vi "6_AC_Akım_Harmonik.vi"(9 "Ölçüm Süresi [sn]":i32=60, 10 "Remote IP Address":string="10.1.21.100") -> (0 "error out":errorcluster, 1 "FD 2":dbl[][](array[numeric]) format="%_5f", 2 "FD 1":dbl[][](array[numeric]) format="%_5f")   [LabVIEW 2014]
panel:
  out "Akım Harmonik FD2 Ich":sgl[][](array[numeric]) format="%_5f"
  out "Akım Harmonik FD2 Ibh":sgl[][](array[numeric]) format="%_5f"
  out "Akım Harmonik FD2 Iah":sgl[][](array[numeric]) format="%_5f"
  in  "Akım Harmonik FD2 Ich Register":u16=1229
  in  "Akım Harmonik FD2 Ibh Register":u16=1129
  in  "Akım Harmonik FD2 Iah Register":u16=1029
  out "Akım Harmonik FD1 Ich":sgl[][](array[numeric]) format="%_5f"
  in  "Akım Harmonik FD1 Ich Register":u16=565
  out "Akım Harmonik FD1 Ibh":sgl[][](array[numeric]) format="%_5f"
  in  "Akım Harmonik FD1 Ibh Register":u16=465
  out "Akım Harmonik FD1 Iah":sgl[][](array[numeric]) format="%.4f"
  out "Numeric":i32
  in  "Akım Harmonik FD1 Iah Register":u16=365
  out "time stamp":timestamp=timestamp(1426515300 s since 1904-01-01) format="%<%H:%M:%S>T"
  in  "Remote Port":u16=1502
  in  "Stop":bool
  # "MB Ethernet Example Master.vi\n\nInstructions\n1. Run MB Ethernet Example Slave.vi\n2. Run this VI.\n3. Modify the discrete inputs or input registers on the slave -> they're updated on the master.\n4. Modify the coils and registers on the master -> they're updated on the slave."
  # "TCP Parameters"
  # "Slave Read-only Registers"
  # "1Har"
  # "1.Har"
  # "2.Har"
  # "3.Har"
  # "4.Har"
  # "5.Har"
  # "6.Har"
  # "7.Har"
  # "8.Har"
  # "9.Har"
  # "10.Har"
  # "2.Har"
  # "3.Har"
  # "4.Har"
  # "1Har"
  # "2.Har"
  # "3.Har"
  # "4.Har"
  # "1.Har"
  # "2.Har"
  # "3.Har"
  # "4.Har"
  # "5.Har"
  # "6.Har"
  # "7.Har"
  # "8.Har"
  # "9.Har"
  # "10.Har"
  # "1Har"
  # "2.Har"
  # "3.Har"
  # "4.Har"
  # "1Har"
  # "2.Har"
  # "3.Har"
  # "4.Har"
  # "1Har"
  # "2.Har"
  # "3.Har"
  # "4.Har"
  # "1Har"
  # "2.Har"
  # "3.Har"
  # "4.Har"
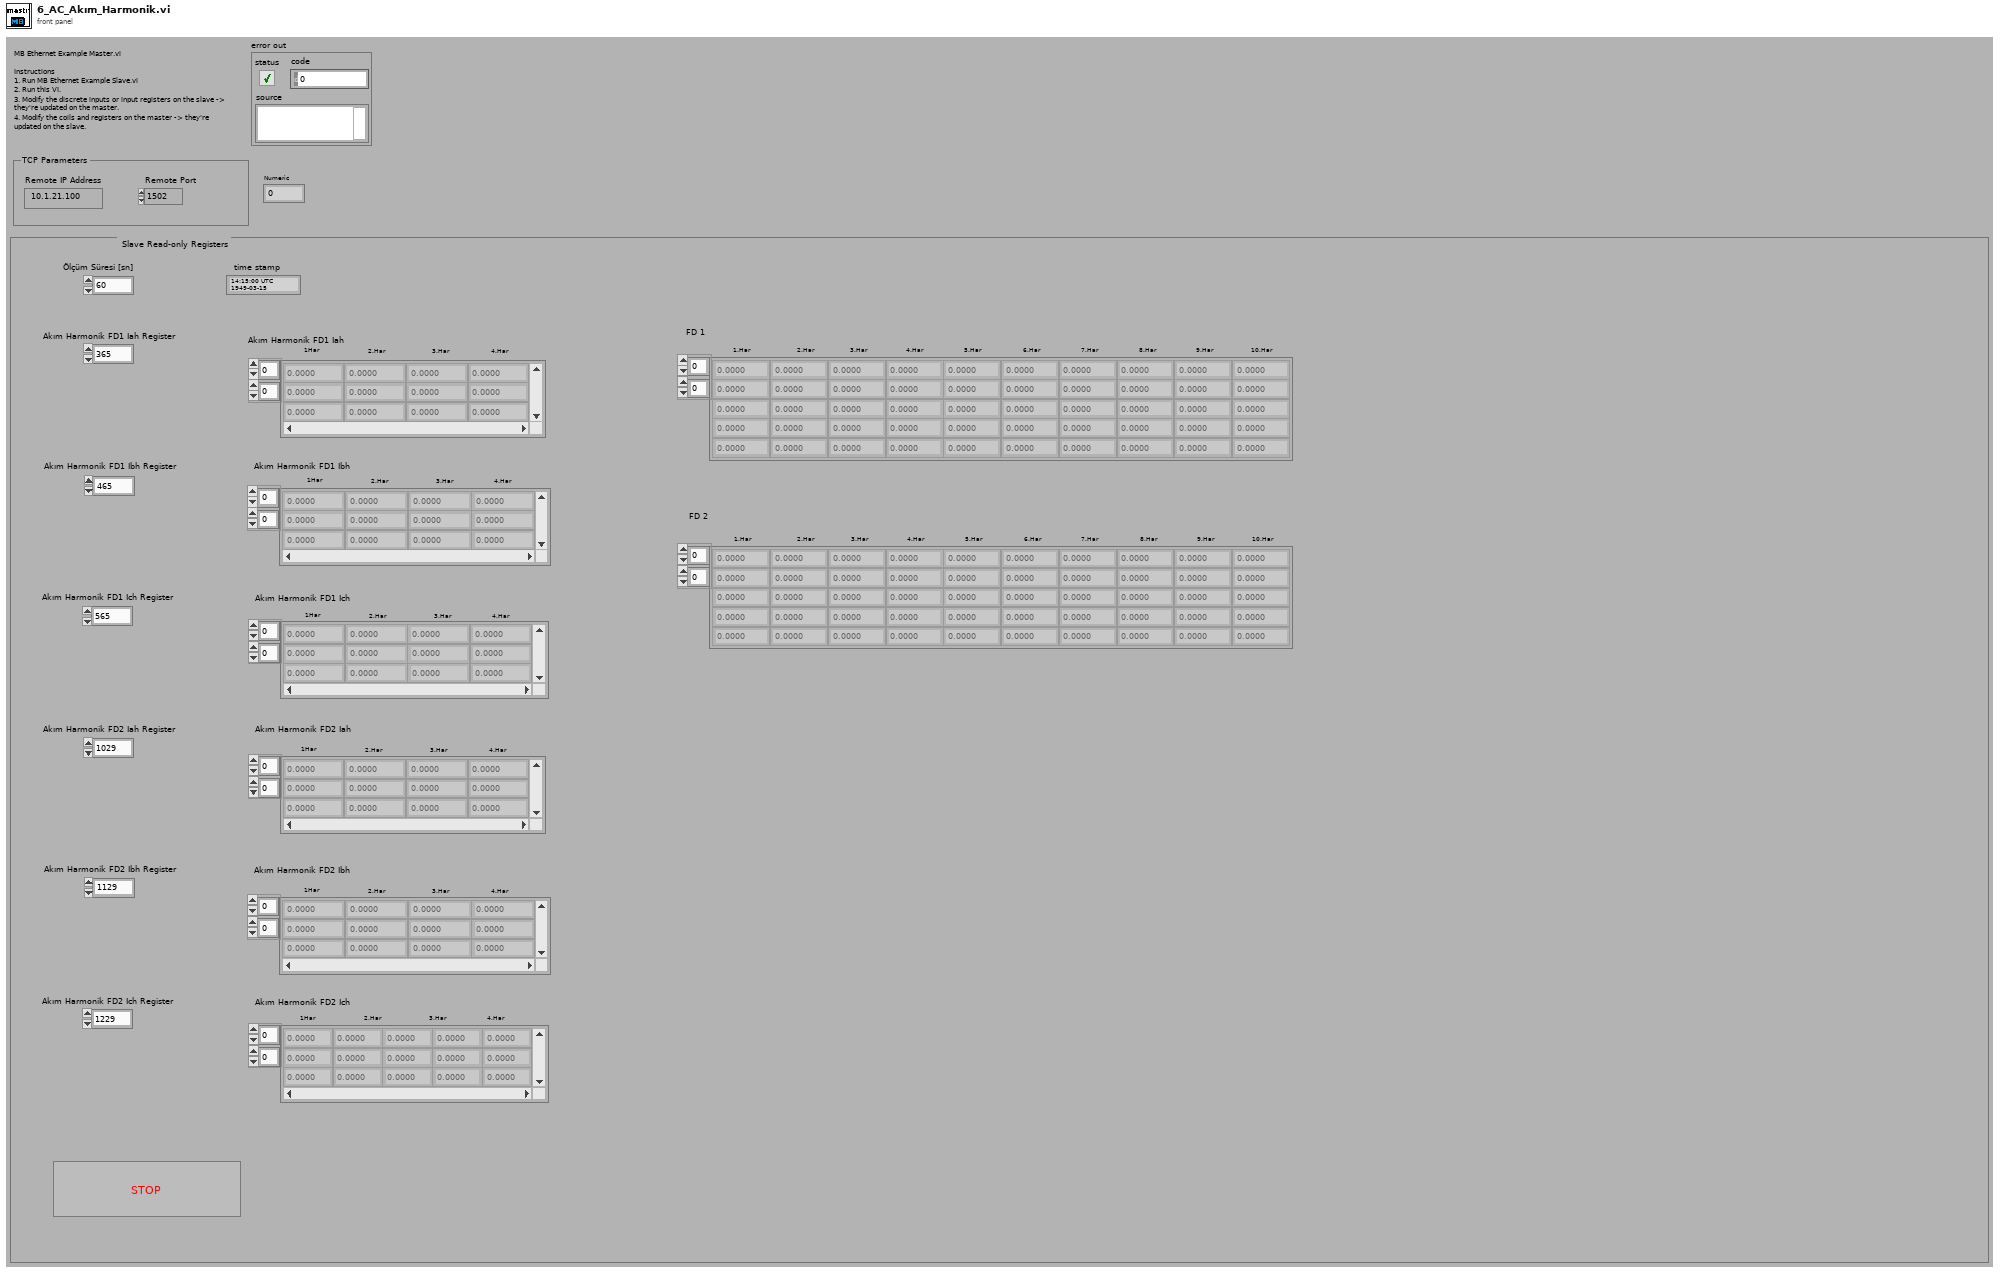
[diagram p1: front panel]
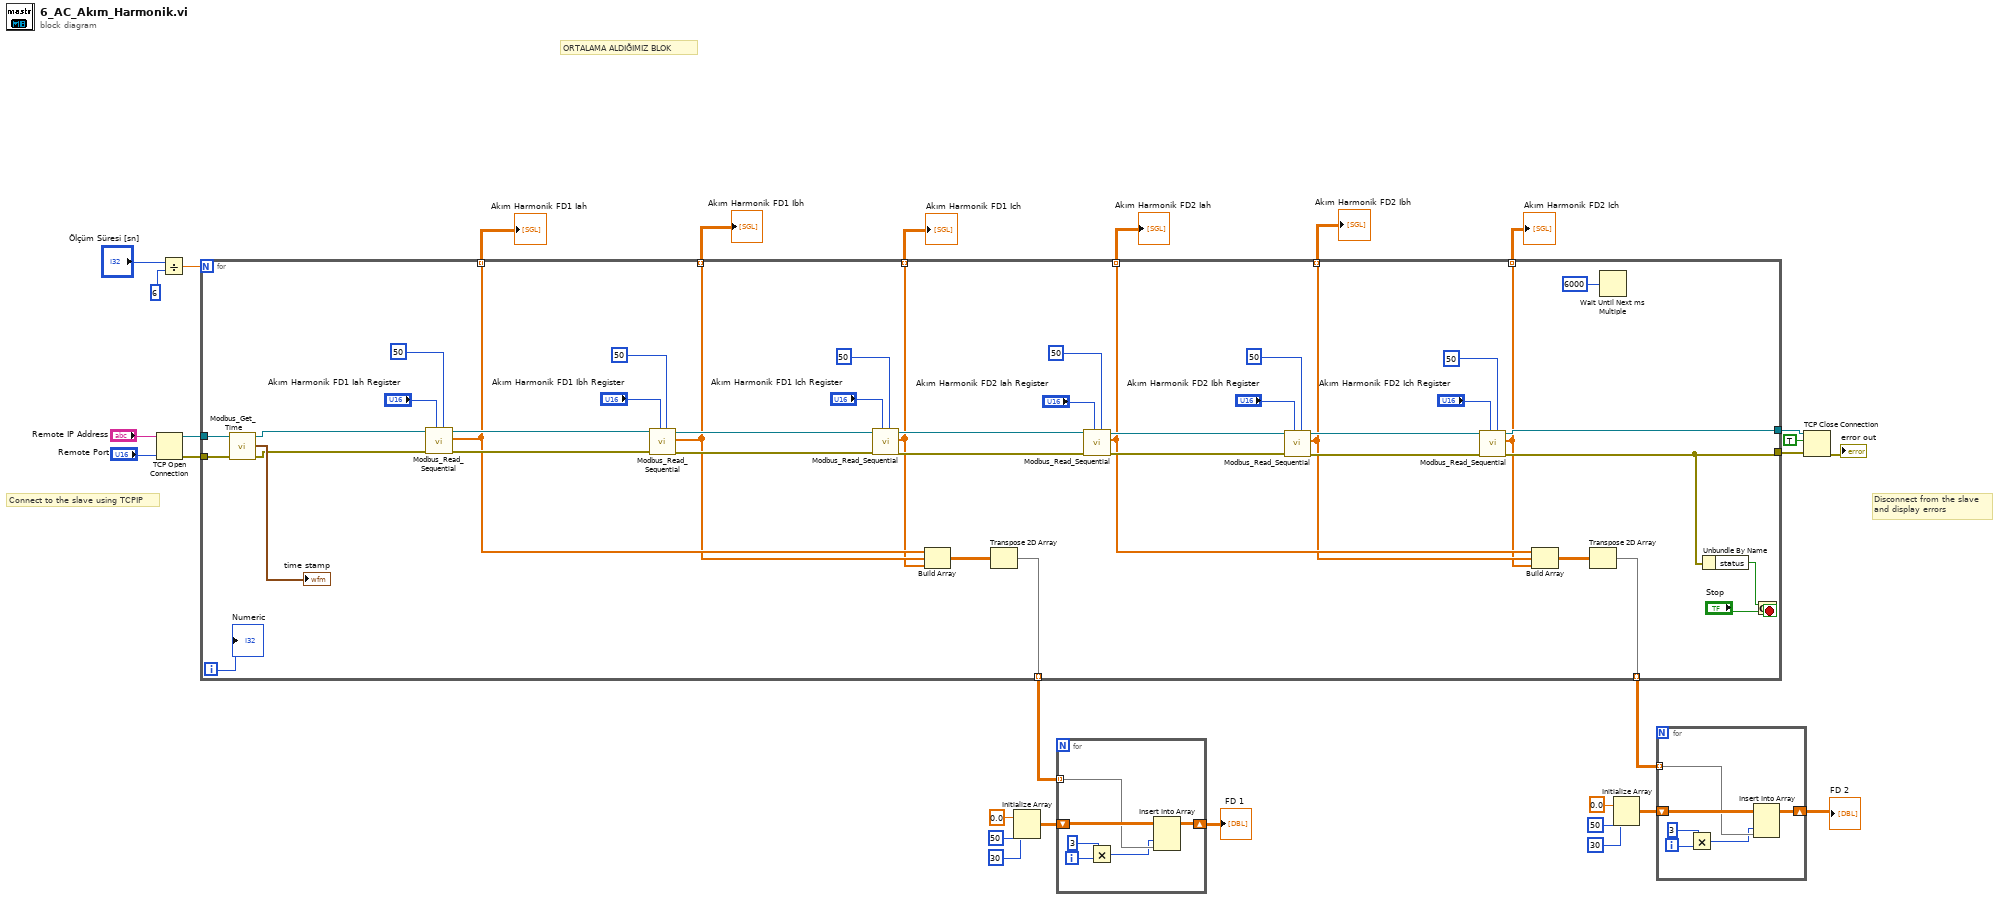
[diagram p0: block diagram]
diagram:
  # "ORTALAMA ALDIĞIMIZ BLOK"
  # "Disconnect from the slave\nand display errors"
  # "Connect to the slave using TCPIP"
  n1 = TCP Open Connection(address="Remote IP Address", remote port or service name="Remote Port") -> (connection ID=w27:refnum<k5>, error out=w26:errorcluster)  [unwired: 1 in, 2 out]
  n2 = Divide(x="Ölçüm Süresi [sn]", y=6) -> (x/y=w23:dbl)
  n3 = for {
    N: w23 -> [_]
    tunnel: w27 -> [w72]
    tunnel: w26 -> [w71]
    tunnel: [w39] -> w20 mode=indexing
    tunnel: [w38] -> w19 mode=indexing
    tunnel: [w37] -> w18 mode=indexing
    tunnel: [w36] -> w17 mode=indexing
    tunnel: [w35] -> w16 mode=indexing
    tunnel: [w34] -> w15 mode=indexing
    tunnel: [w41] -> w14
    tunnel: [w40] -> w13
    tunnel: [w31] -> w12 mode=indexing
    tunnel: [w30] -> w2 mode=indexing
    i -> [w66]
    stop <- w67 stop-if-true
    n4 = call "Modbus_Get_Time.vi"("error in (no error)"=w71, "TCP Network Connection in"=w72) -> ("error out"=w68:errorcluster, "Time Stamp"=→"time stamp":timestamp, "TCP Network Connection out"=w69:refnum<k5>)  [unwired: 6 in, 1 out]
    n5 = call "Modbus_Read_Sequential.vi"("Number of Elements"=50, "Start Address"="Akım Harmonik FD1 Iah Register", "error in (no error)"=w68, "TCP Network Connection in"=w69) -> ("error out"=w62:errorcluster, "Array of Elements (RMS)"=w39:sgl[], "TCP Network Connection out"=w63:refnum<k5>)  [unwired: 5 in]
    n6 = call "Modbus_Read_Sequential.vi"("Number of Elements"=50, "Start Address"="Akım Harmonik FD1 Ibh Register", "error in (no error)"=w62, "TCP Network Connection in"=w63) -> ("error out"=w55:errorcluster, "Array of Elements (RMS)"=w38:sgl[], "TCP Network Connection out"=w54:refnum<k5>)  [unwired: 5 in]
    n7 = call "Modbus_Read_Sequential.vi"("Number of Elements"=50, "Start Address"="Akım Harmonik FD1 Ich Register", "error in (no error)"=w55, "TCP Network Connection in"=w54) -> ("error out"=w43:errorcluster, "Array of Elements (RMS)"=w37:sgl[], "TCP Network Connection out"=w42:refnum<k5>)  [unwired: 5 in]
    n8 = Build Array(w39, w38, w37) -> (w32:sgl[][])
    n9 = Transpose 2D Array(2D array=w32) -> (transposed array=w31:sgl[][])
    n10 = call "Modbus_Read_Sequential.vi"("Number of Elements"=50, "Start Address"="Akım Harmonik FD2 Iah Register", "error in (no error)"=w43, "TCP Network Connection in"=w42) -> ("error out"=w52:errorcluster, "Array of Elements (RMS)"=w36:sgl[], "TCP Network Connection out"=w53:refnum<k5>)  [unwired: 5 in]
    n11 = call "Modbus_Read_Sequential.vi"("Number of Elements"=50, "Start Address"="Akım Harmonik FD2 Ibh Register", "error in (no error)"=w52, "TCP Network Connection in"=w53) -> ("error out"=w45:errorcluster, "Array of Elements (RMS)"=w35:sgl[], "TCP Network Connection out"=w44:refnum<k5>)  [unwired: 5 in]
    n12 = call "Modbus_Read_Sequential.vi"("Number of Elements"=50, "Start Address"="Akım Harmonik FD2 Ich Register", "error in (no error)"=w45, "TCP Network Connection in"=w44) -> ("error out"=w41:errorcluster, "Array of Elements (RMS)"=w34:sgl[], "TCP Network Connection out"=w40:refnum<k5>)  [unwired: 5 in]
    n13 = Build Array(w36, w35, w34) -> (w33:sgl[][])
    n14 = Transpose 2D Array(2D array=w33) -> (transposed array=w30:sgl[][])
    n15 = Wait Until Next ms Multiple(millisecond multiple=u32 6000) -> ()  [unwired: 1 out]
    n16 = Unbundle By Name(w41) -> ("status"=w64:bool)
    n17 = Or(x=w64, y="Stop") -> (x .or. y?=w67:bool)
    "Numeric" <- w66
  }
  "Akım Harmonik FD1 Iah" <- w20
  "Akım Harmonik FD1 Ibh" <- w19
  "Akım Harmonik FD1 Ich" <- w18
  "Akım Harmonik FD2 Iah" <- w17
  "Akım Harmonik FD2 Ibh" <- w16
  "Akım Harmonik FD2 Ich" <- w15
  n18 = Initialize Array(0.0 ("element"), 50 ("dimension size"), 30 ("dimension size")) -> (w8:dbl[][])
  n19 = for {
    tunnel: w12 -> [w77] mode=indexing
    shift-right: [w78] -> w7
    shift-left: w8 -> [w79]
    i -> [w76]
    n20 = Multiply(x=3, y=w76) -> (x*y=w74:i32)
    n21 = Insert Into Array(array=w79, index (col)=w74, new element=w77) -> (w78:dbl[][])  [unwired: 1 in]
  }
  "FD 1" <- w7
  n22 = Initialize Array(0.0 ("element"), 50 ("dimension size"), 30 ("dimension size")) -> (w3:dbl[][])
  n23 = for {
    tunnel: w2 -> [w83] mode=indexing
    shift-right: [w84] -> w1
    shift-left: w3 -> [w85]
    i -> [w82]
    n24 = Multiply(x=3, y=w82) -> (x*y=w80:i32)
    n25 = Insert Into Array(array=w85, index (col)=w80, new element=w83) -> (w84:dbl[][])  [unwired: 1 in]
  }
  "FD 2" <- w1
  n26 = TCP Close Connection(connection ID=w13, abort (F)=TRUE, error in (no error)=w14) -> (error out=→"error out":errorcluster)  [unwired: 1 out]
